vi "Instr_InitObject.vi"(8 "error in (no error)":errorcluster, 9 "Instrument Configuration":variant, 10 "Instrument address":refnum<visa-resource-name>, 11 "KE487 in":refnum<class "KE487.lvclass">) -> (0 "error out":errorcluster, 3 "KE487 out":refnum<class "KE487.lvclass">)   [LabVIEW 2013, in "KE487.lvclass"]
uses:
  KE487.lvclass
  KE487_CommandsGlobal.vi
  SupplyControl.lvclass
  InstrumentSetup.vi
  InstrControl.lvclass
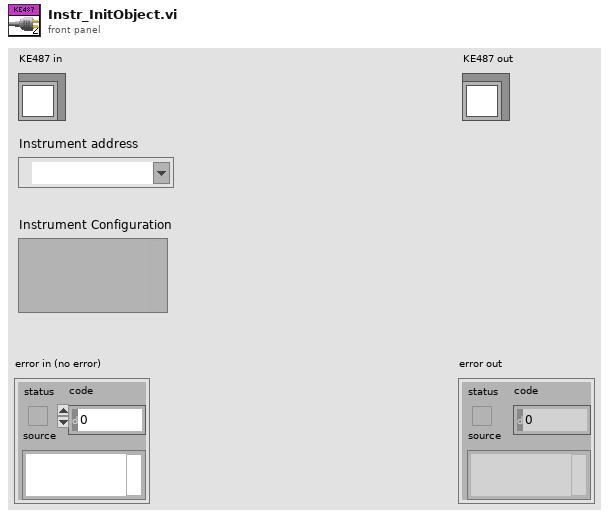
[diagram p1: front panel]
types:
  T1 = cluster{"Compliance":u16, "Range:":u16, "KE487":refnum<class "KE487.lvclass">}
  T2 = cluster{"Instrument name":string, "Command \"Reset\"":string, "Command \"Initialise\"":string, "Command \"Arm\"":string, "Command \"SetVolts\"":string, "Command \"Compliance?\"":string, "Command \"Standby\"":string, "Command \"Read Current\"":string}
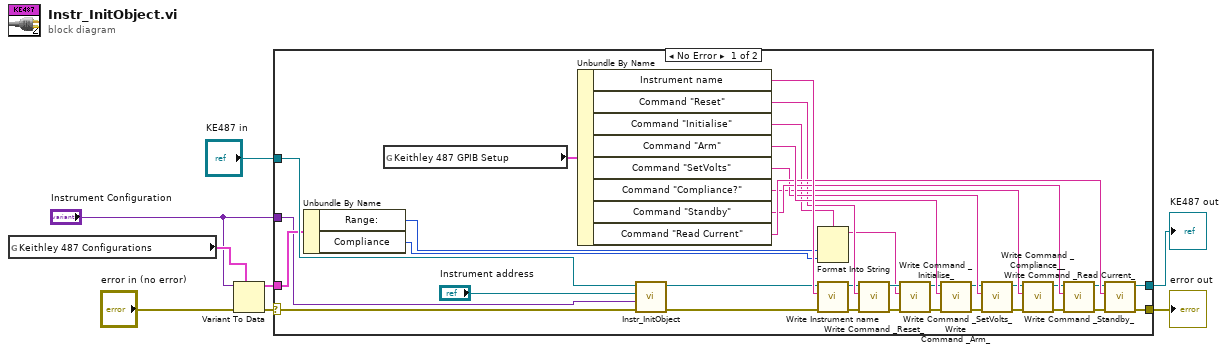
[diagram p0: block diagram]
diagram:
  n1 = global read "InstrumentSetup.vi" "Keithley 487 Configurations"() -> (w5:T1)
  n2 = Variant To Data(error in="error in (no error)", type=w5, Variant="Instrument Configuration") -> (data=w1:T1, error out=w2:errorcluster)
  n3 = case shown="No Error" w2 {
    selector: w2 -> [w11 w45]
    tunnel: [w23 w45] -> w6
    tunnel: [w24 w44] -> w7
    tunnel: "KE487 in" -> [w12 w44]
    tunnel: w1 -> [w10 _]
    tunnel: "Instrument Configuration" -> [w9 _]
    frame No Error {
      n4 = Unbundle By Name(w10) -> ("Range:"=w22:u16, "Compliance"=w19:u16)
      n5 = global read "KE487_CommandsGlobal.vi" "Keithley 487 GPIB Setup"() -> (w18:T2)
      n6 = Unbundle By Name(w18) -> ("Instrument name"=w43:string, "Command \"Reset\""=w37:string, "Command \"Initialise\""=w21:string, "Command \"Arm\""=w42:string, "Command \"SetVolts\""=w39:string, "Command \"Compliance?\""=w38:string, "Command \"Standby\""=w40:string, "Command \"Read Current\""=w41:string)
      n7 = call-parent "Instr_InitObject.vi"("error in (no error)"=w11, "Instrument Configuration"=w9, "Instrument address"="Instrument address", "SupplyControl in"=w12) -> ("error out"=w14:errorcluster, "SupplyControl out"=w15:refnum<class "KE487.lvclass">)  [unwired: 6 in]
      n8 = Format Into String(format string=w21, w22, w19) -> (resulting string=w20:string)  [unwired: 2 in, 1 out]
      n9 = call-dynamic "Write Instrument name.vi"("error in (no error)"=w14, "Instrument name"=w43, "InstControl in"=w15) -> ("error out"=w16:errorcluster, "InstControl out"=w17:refnum<class "KE487.lvclass">)  [unwired: 7 in]
      n10 = call-dynamic "Write Command _Reset_.vi"("error in (no error)"=w16, "Command \"Reset\""=w37, "SupplyControl in"=w17) -> ("error out"=w30:errorcluster, "SupplyControl out"=w36:refnum<class "KE487.lvclass">)  [unwired: 7 in]
      n11 = call-dynamic "Write Command _Initialise_.vi"("error in (no error)"=w30, "Command \"Initialise\""=w20, "SupplyControl in"=w36) -> ("error out"=w29:errorcluster, "SupplyControl out"=w35:refnum<class "KE487.lvclass">)  [unwired: 7 in]
      n12 = call-dynamic "Write Command _Arm_.vi"("error in (no error)"=w29, "Command \"Arm\""=w42, "SupplyControl in"=w35) -> ("error out"=w28:errorcluster, "SupplyControl out"=w34:refnum<class "KE487.lvclass">)  [unwired: 7 in]
      n13 = call-dynamic "Write Command _SetVolts_.vi"("error in (no error)"=w28, "Command \"SetVolts\""=w39, "SupplyControl in"=w34) -> ("error out"=w27:errorcluster, "SupplyControl out"=w33:refnum<class "KE487.lvclass">)  [unwired: 7 in]
      n14 = call-dynamic "Write Command _Compliance__.vi"("error in (no error)"=w27, "Command \"Compliance?\""=w38, "SupplyControl in"=w33) -> ("error out"=w26:errorcluster, "SupplyControl out"=w32:refnum<class "KE487.lvclass">)  [unwired: 7 in]
      n15 = call-dynamic "Write Command _Standby_.vi"("error in (no error)"=w26, "Command \"Standby\""=w40, "SupplyControl in"=w32) -> ("error out"=w25:errorcluster, "SupplyControl out"=w31:refnum<class "KE487.lvclass">)  [unwired: 7 in]
      n16 = call-dynamic "Write Command _Read Current_.vi"("error in (no error)"=w25, "Command \"Read Current\""=w41, "SupplyControl in"=w31) -> ("error out"=w23:errorcluster, "SupplyControl out"=w24:refnum<class "KE487.lvclass">)  [unwired: 7 in]
    }
    frame Error {
    }
  }
  "error out" <- w6
  "KE487 out" <- w7
